vi "CAPTH Main Panel.vi"(11 "Expt State In":T2) -> (3 "Expt State Out":T2)   [LabVIEW 2020]
uses:
  CFTS Main Panel SubVIs/CFTS-Experiment State.ctl
  Typedefs/CAPTH-State.ctl
  CFTS Main Panel SubVIs/CFTS-Data Type Enum.ctl
panel:
  out "validate save history":bool
  out "XY Graph":cluster{"X":dbl, "Y":dbl}[](graph)
  out "finished":errorcluster
  in  "NOTES":string
  out "exit signal":bool
  in  "Analysis":bool
  in  "Response":T1={"Averages (3dB steps)"=12, "Time Window (ms)"=8.5, "dt (ms)"=10.0, "Grass gain"=1000.0, "CRITERION (uV)"=5.0, "CEILING (dB atten)"=6.0, "Use previous"=FALSE, "Save avgs"=FALSE, "Save raw"=FALSE, "Save history"=FALSE, "CEILING (dB SPL)"=6.0} {"CRITERION (uV)" format="%.2f"; "Time Window (ms)" format="%.2f"}
  out "User":string
  out "Run #":u16=14
  out "ID #":u16=1
  out "ave 2":cluster{i32, dbl, ext[]}(graph)={0, 0.01, []}
  in  "Stimulus":T3={" EAR"=enum."LEFT\n", "HI FREQ"=10.0, "LO FREQ"=2.5, "Steps/octave"=1, "Rep Rate (/s)"=20.0, "Alternate Polarity"=FALSE, "# CYCLES"=1, "Duration (ms)"=0.0, "Ramp (ms)"=0.0}
  in  "RETURN":bool
  in  "START":bool
  out "POST-EXPOSURE TIME (sec)":u32
  out "kHz":dbl=0.25 caption="Current frequency (kHz)" format="%.2f"
  out "Averages (1dB steps)":i32=24
  out "dB SPL 2":i32=20
  out "dB SPL 1":i32=74
  out "CYCLE":i32=1
  out "AUDIOGRAM":cluster{"Freq":dbl[], "Threshold":dbl[]}[](graph)
  out "ave 1":cluster{i32, dbl, ext[]}(graph)={0, 0.01, []}
  in  "STOP":bool
  # "Stimulus"
  # "1 dB per step"
  # "3 dB per step"
  # "Response"
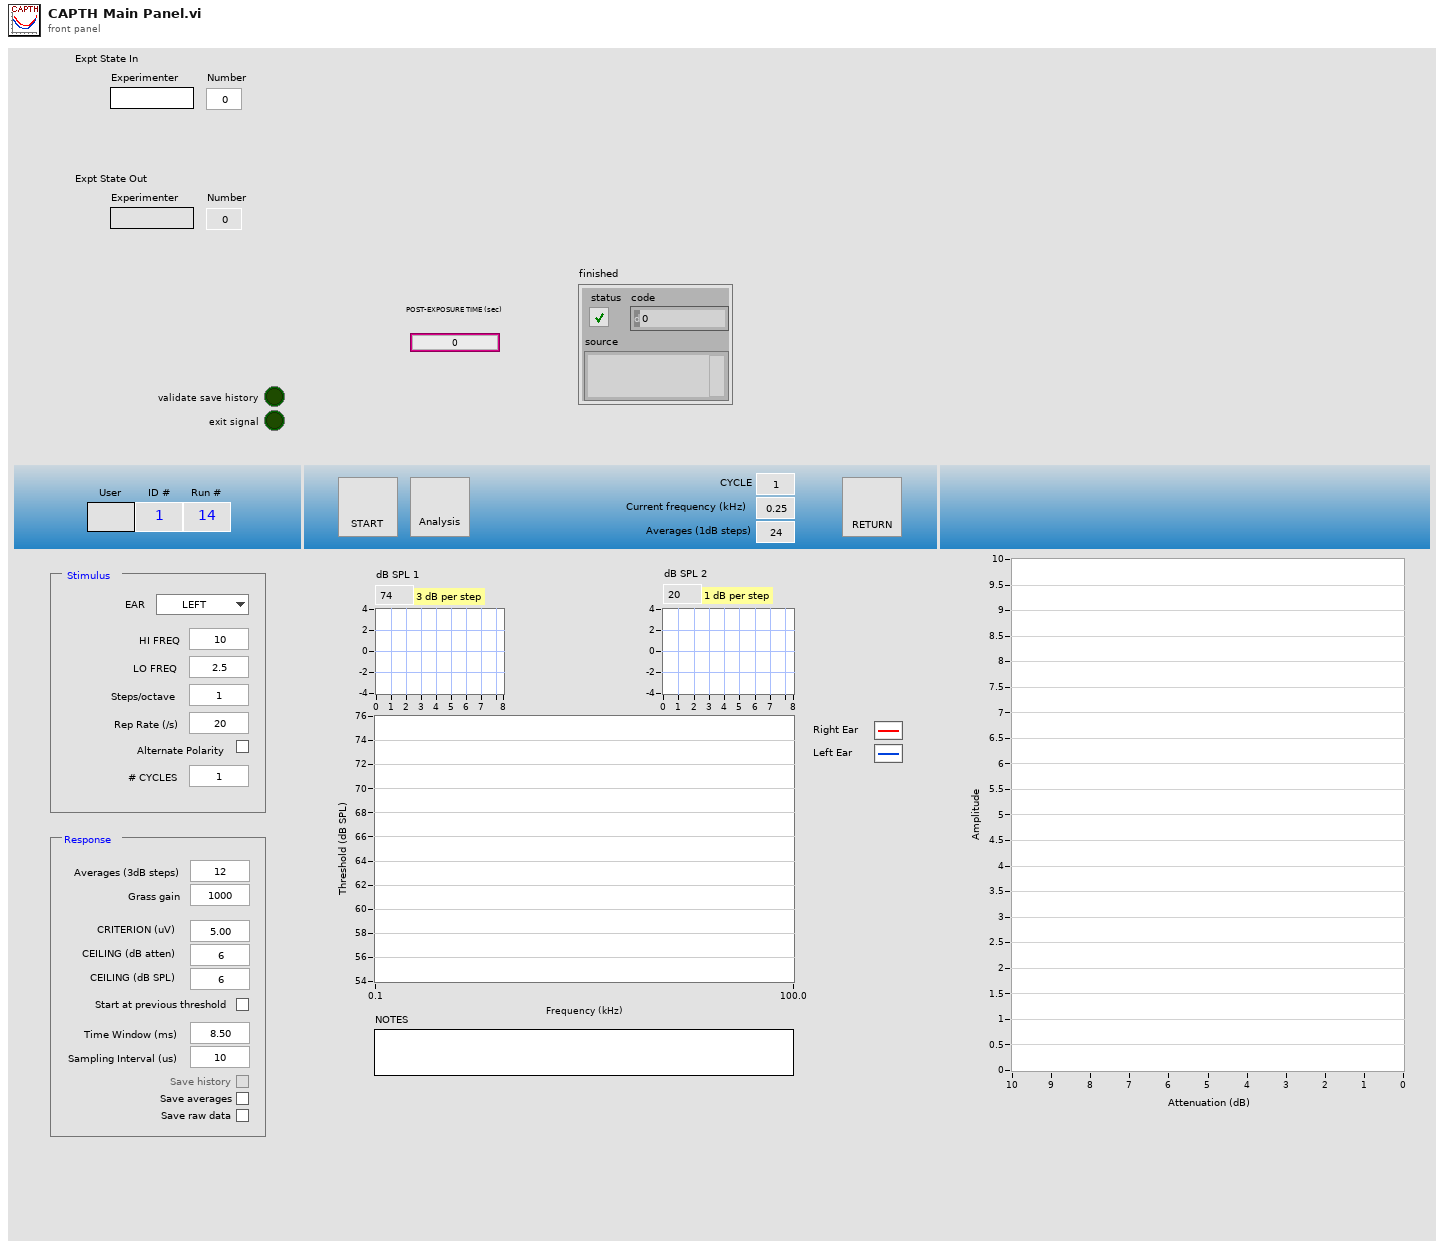
[diagram p1: front panel]
types:
  T1 = cluster{"Averages (3dB steps)":i32, "Time Window (ms)":dbl, "dt (ms)":dbl, "Grass gain":dbl, "CRITERION (uV)":dbl, "CEILING (dB atten)":dbl, "Use previous":bool, "Save avgs":bool, "Save raw":bool, "Save history":bool, "CEILING (dB SPL)":dbl}
  T2 = typedef "CFTS-Experiment State.ctl" = cluster{"Experimenter":string, "Number":u32, "Right":string, "Left":string, "Data Folder":path, "State File":path, "Version Info":string, "End Exposure Time":dbl, "Exposure Duration":string, "Run #":cluster{"CAP":i16, "ABR":i16, "DP":i16, "VsEP":i16, "MeasSeq":i16, "SubSeq":i16, "SFOAE":i16}}
  T3 = cluster{" EAR":enum16{"RIGHT", "LEFT\n", "ALTERNATE"}, "HI FREQ":dbl, "LO FREQ":dbl, "Steps/octave":u8, "Rep Rate (/s)":dbl, "Alternate Polarity":bool, "# CYCLES":u8, "Duration (ms)":dbl, "Ramp (ms)":dbl}
  T4 = typedef "CAPTH-IPC.ctl" = cluster{"Start":refnum<notifier>, "Control":refnum<notifier>, "Analysis":refnum<queue>}
  T5 = typedef "CAPTH-State.ctl" = cluster{"Datafile":path, "running":bool, "user":string, "aborted":bool}
  T6 = typedef "CFTS-Data Type Enum.ctl" = enum16{"CAP", "ABR", "DP", "VsEP", "MeasSeq", "SFOAE"}
  T7 = enum8{"Enabled", "Disabled", "Disabled and Grayed Out"}
  T8 = typedef "CAPTH-Parameters.ctl" = cluster{"Stimulus":T9, "Response":T10}
  T9 = typedef "CAPTH-Stimulus.ctl" = cluster{"EAR":enum16{"RIGHT", "LEFT\n", "ALTERNATE"}, "HI FREQ":dbl, "LO FREQ":dbl, "FREQ STEP":u8, "Rep Rate (/s)":dbl, "Alternate Polarity":bool, "# CYCLES":u8, "Duration (ms)":dbl, "Ramp (ms)":dbl}
  T10 = typedef "CAPTH-Response.ctl" = cluster{"Averages (3dB steps)":i32, "Time Window (ms)":dbl, "dt (us)":dbl, "Grass gain":dbl, "CRITERION (mV)":dbl, "CEILING (dB atten)":dbl, "Use previous":bool, "Save avgs":bool, "Save raw":bool, "Save history":bool, "CEILING (dB SPL)":dbl}
  T11 = cluster{"Freq":dbl[], "Threshold SPL":dbl[], "Max SPL":dbl[]}[]
  T12 = cluster{"Datafile path":path, "Params":T8, "data":cluster{"Freq":dbl[], "Threshold SPL":dbl[], "Max SPL":dbl[]}[]}
  T13 = typedef "CAPTH-Start Data.ctl" = cluster{"Datafile":path, "Params":T8, "data":cluster{"Freq":dbl[], "Threshold atten":dbl[], "Max SPL":dbl[]}[]}
  T14 = cluster{"Freq":dbl[], "Threshold atten":dbl[], "Max SPL":dbl[]}[]
  T15 = typedef "CAPTH-Runtime.ctl" = cluster{"Sampling rate":dbl, "AO npts":i32, "Alternate Polarity":bool, "AI npts":i32, "Npts window":i32, "1dB avgs":i32, "Datafile":path}
  T16 = typedef "CAPTH-StimCon.ctl" = cluster{"ear":i32, "freq":i32, "Max SPL":dbl}
  T17 = cluster{"Freq":dbl[], "Threshold":dbl[], "Max SPL":dbl[]}[]
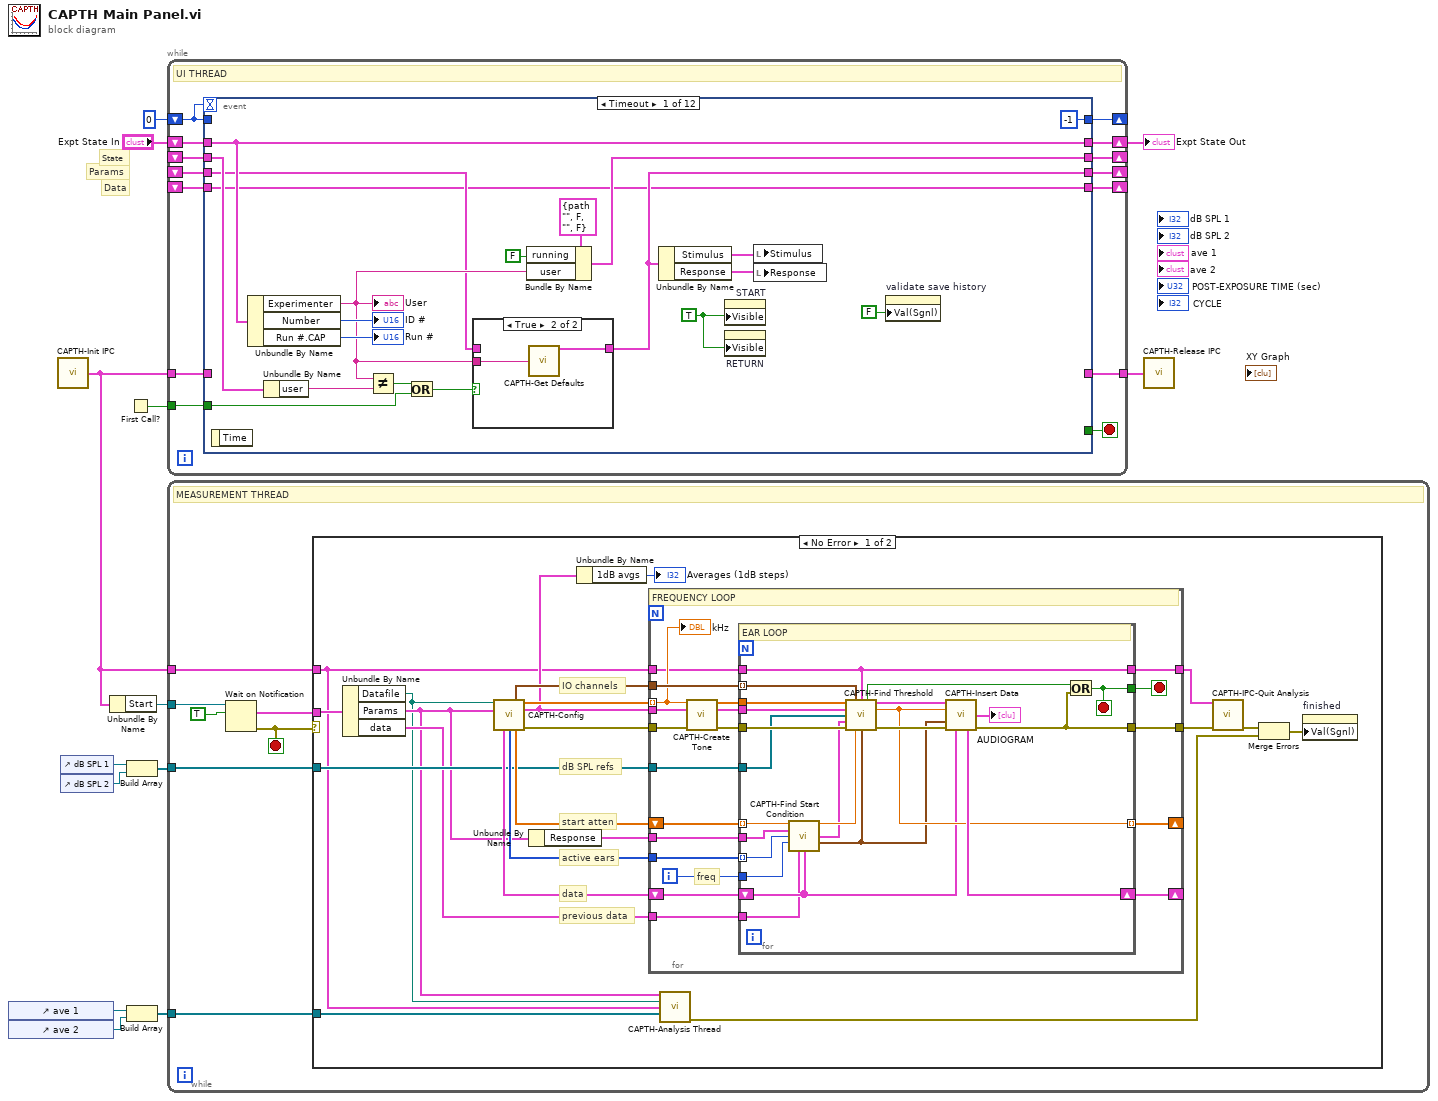
[diagram p0: block diagram]
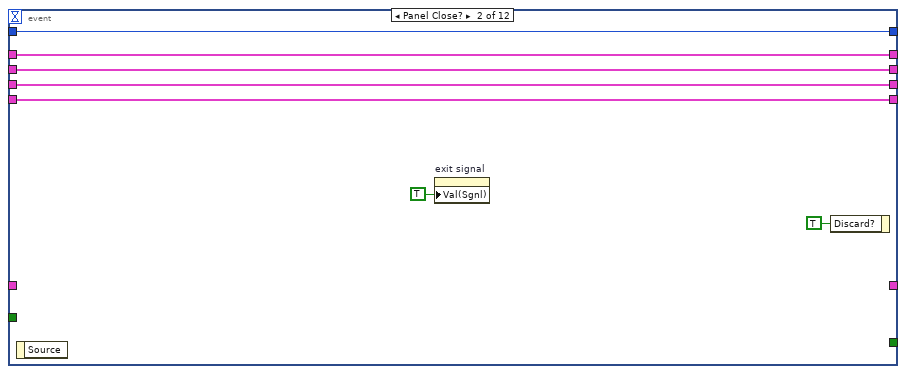
[diagram p4: hidden frame]
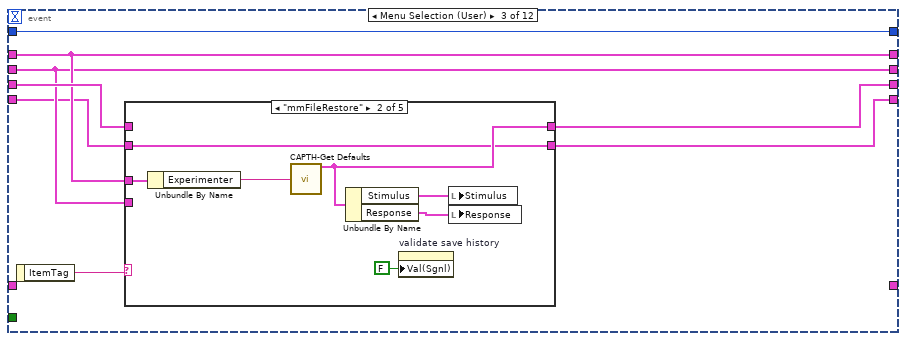
[diagram p5: hidden frame]
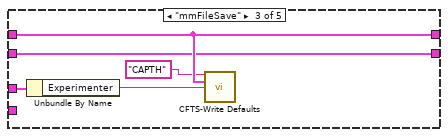
[diagram p7: hidden frame]
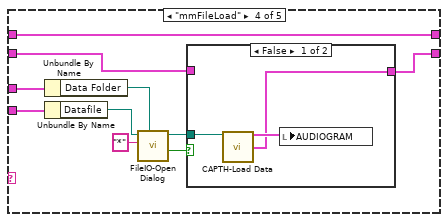
[diagram p8: hidden frame]
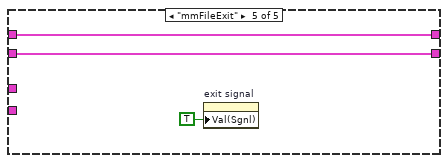
[diagram p10: hidden frame]
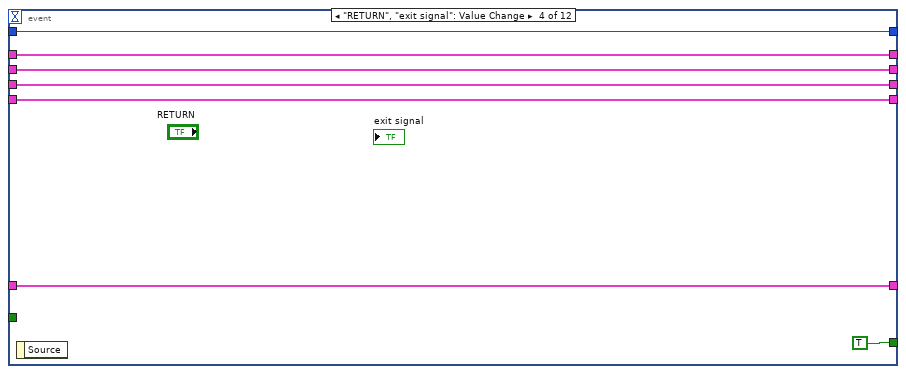
[diagram p11: hidden frame]
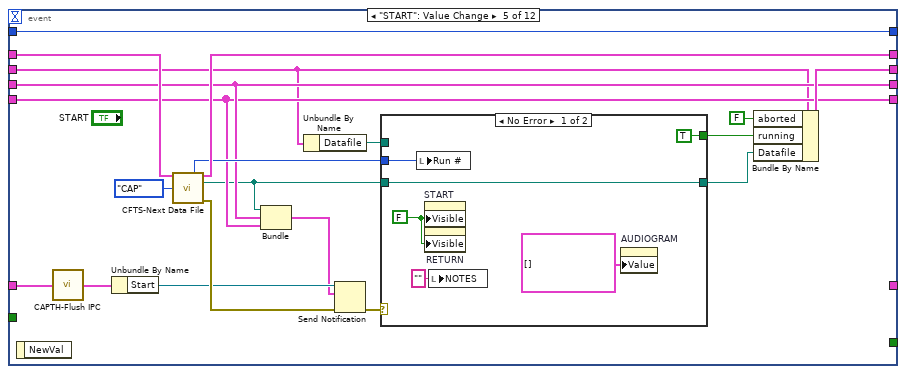
[diagram p12: hidden frame]
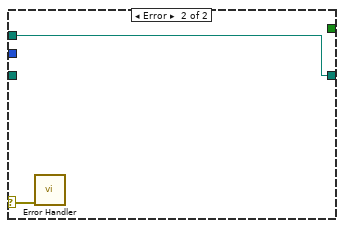
[diagram p13: hidden frame]
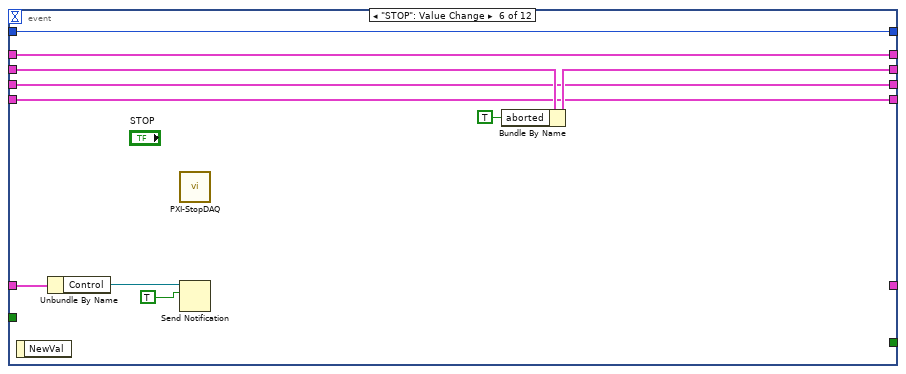
[diagram p14: hidden frame]
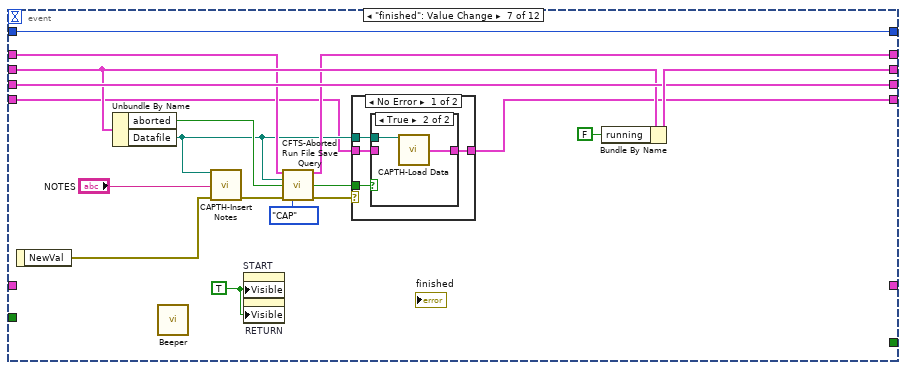
[diagram p15: hidden frame]
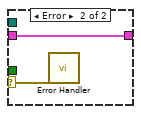
[diagram p17: hidden frame]
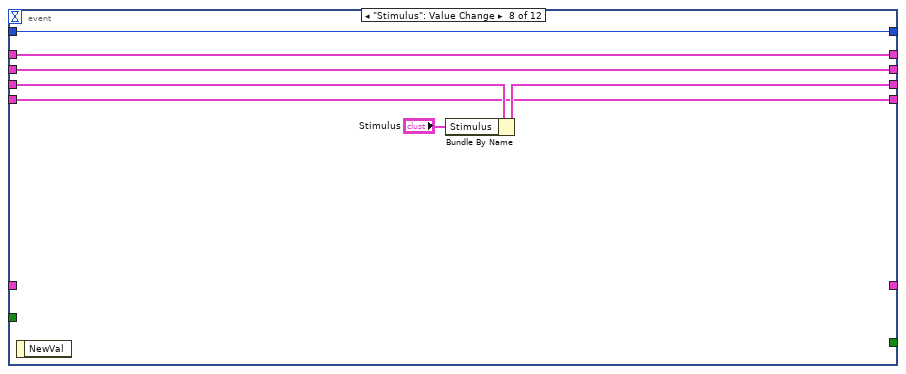
[diagram p18: hidden frame]
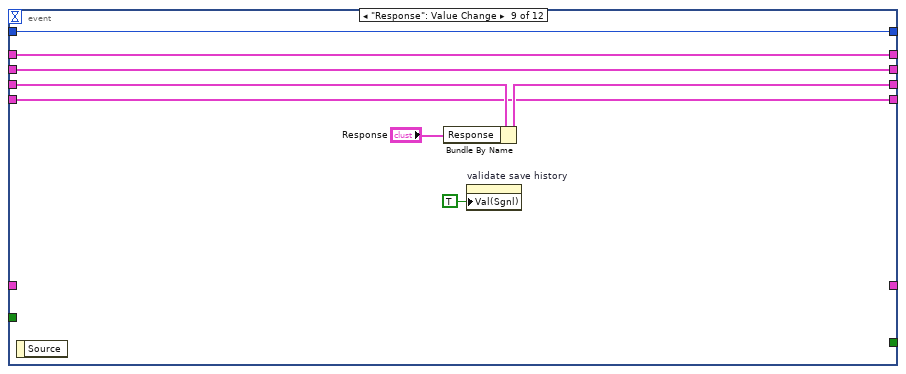
[diagram p19: hidden frame]
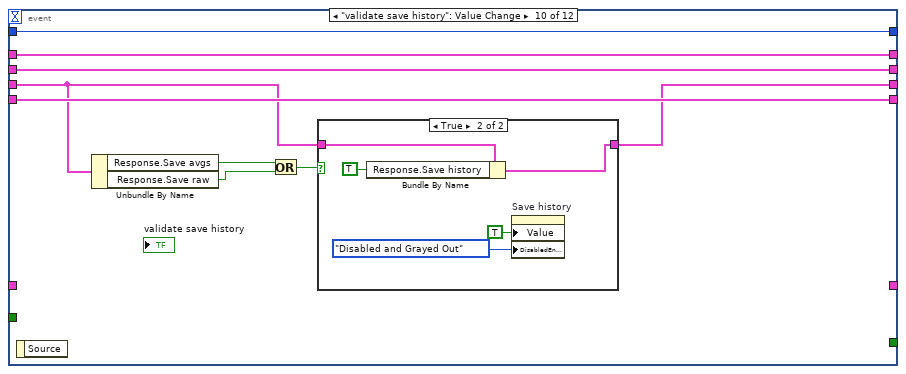
[diagram p20: hidden frame]
diagram:
  # "Data"
  # "Params"
  # "State"
  n1 = control-ref of="ave 1"() -> (w3:refnum<vi>)
  n2 = control-ref of="ave 2"() -> (w2:refnum<vi>)
  n3 = call "CAPTH-Init IPC.vi"() -> ("IPC"=w5:T4)  [unwired: 15 in]
  n4 = control-ref of="dB SPL 1"() -> (w10:refnum<vi>)
  n5 = control-ref of="dB SPL 2"() -> (w9:refnum<vi>)
  n6 = Unbundle By Name(w5) -> ("Start"=w7:refnum<notifier>)
  n7 = First Call?() -> (First Call?: T/F=w12:bool)
  n8 = Build Array(w10, w9) -> (w4:refnum<vi>[])
  n9 = Build Array(w3, w2) -> (w1:refnum<vi>[])
  n10 = while {
    tunnel: w5 -> [w27]
    shift-right: [w25] -> _
    shift-left: 0 -> [w21]
    tunnel: [w24] -> w6
    tunnel: w12 -> [w23]
    shift-right: [w20] -> w8
    shift-left: "Expt State In" -> [w22]
    shift-right: [w19] -> _
    shift-left: _ -> [w18]
    shift-right: [w16] -> _
    shift-left: _ -> [w17]
    shift-right: [w15] -> _
    shift-left: _ -> [w14]
    stop <- w26 stop-if-true
    # "UI THREAD"
    n11 = event shown="[0] Timeout" {
      selector: _ -> [_ _ _ _ _ _ _ _ _ _ _ _]
      dyn-events: _ -> [_ _ _ _ _ _ _ _ _ _ _ _]
      timeout: w21 -> [_ _ _ _ _ _ _ _ _ _ _ _]
      tunnel: w27 -> [_ _ _ w102 w109 w134 _ _ _ _ _ _]
      tunnel: [_ _ _ TRUE _ _ _ _ _ _ _ _] -> w26
      tunnel: [-1 w55 w64 w101 w123 w141 w159 w175 w183 w192 w206 w225] -> w25
      tunnel: [_ _ _ w102 _ _ _ _ _ _ _ _] -> w24
      tunnel: w23 -> [w41 _ _ _ _ _ _ _ _ _ _ _]
      tunnel: w22 -> [w40 w54 w61 w100 w119 w140 w147 w174 w182 w191 w205 w223]
      tunnel: w21 -> [_ w55 w64 w101 w123 w141 w159 w175 w183 w192 w206 w225]
      tunnel: [w40 w54 w61 w100 w118 w140 w146 w174 w182 w191 w205 w223] -> w20
      tunnel: [w39 w53 w60 w99 w122 w138 w157 w173 w181 w190 w204 w224] -> w19
      tunnel: w18 -> [w36 w53 w60 w99 w105 w139 w151 w173 w181 w190 w204 w224]
      tunnel: w17 -> [w33 w52 w62 w98 w113 w136 w155 w172 w180 w185 w202 w220]
      tunnel: [w32 w52 w63 w98 w113 w136 w155 w171 w179 w184 w202 w220] -> w16
      tunnel: [w29 w51 w59 w97 w112 w135 w144 w169 w177 w189 w201 w219] -> w15
      tunnel: w14 -> [w29 w51 w58 w97 w112 w135 w143 w169 w177 w189 w201 w219]
      event Timeout {
        w46 = TRUE ("Visible")
        n12 = event-data() -> ()  [unwired: 1 in, 1 out]
        n13 = Unbundle By Name(w40) -> ("Experimenter"=w37:string, "Number"=→"ID #":u32, "Run #.CAP"=→"Run #":i16)
        "User" <- w37
        n14 = Unbundle By Name(w36) -> ("user"=w35:string)
        n15 = Not Equal?(x=w37, y=w35) -> (x != y?=w43:bool)
        n16 = Or(x=w43, y=w41) -> (x .or. y?=w42:bool)
        n17 = case shown="True" w42 {
          tunnel: w37 -> [_ w49]
          tunnel: w33 -> [w48 _]
          tunnel: [w48 w50] -> w32
          frame False {
          }
          frame True {
            n18 = call "CAPTH-Get Defaults.vi"("User"=w49) -> ("Params"=w50:T8)  [unwired: 14 in]
          }
        }
        n19 = Bundle By Name(cluster=T5 {"Datafile"=path "", "running"=FALSE, "user"="", "aborted"=FALSE} ("State"), "running"=FALSE, "user"=w37) -> (w39:T5)
        n20 = Unbundle By Name(w32) -> ("Stimulus"=w31:T9, "Response"=w30:T10)
        n21 = property on="START" class="Bool"("Visible"=w46) -> ()  [unwired: 2 in, 2 out]
        n22 = property on="RETURN" class="Bool"("Visible"=w46) -> ()  [unwired: 2 in, 2 out]
        n23 = local write "Stimulus"(w31) -> ()
        n24 = local write "Response"(w30) -> ()
        n25 = property on="validate save history" class="Bool (strict)"("Val(Sgnl)"=FALSE ("Value (Signaling)")) -> ()  [unwired: 2 in, 2 out]
      }
      event Panel Close? {
        n26 = event-data() -> ()  [unwired: 1 in, 1 out]
        n27 = property on="exit signal" class="Bool (strict)"("Val(Sgnl)"=TRUE ("Value (Signaling)")) -> ()  [unwired: 2 in, 2 out]
        n28 = event-data("Discard?"=TRUE) -> ()  [unwired: 1 in, 1 out]
      }
      event Menu Selection (User) {
        n29 = event-data() -> ("ItemTag"=w65:string)  [unwired: 1 in]
        n30 = case shown="\"mmFileRestore\"" w65 {
          tunnel: w60 -> [_ _ _ w84 _]
          tunnel: [w67 w72 w77 w82 w95] -> w63
          tunnel: w62 -> [w67 _ w77 w82 w95]
          tunnel: w61 -> [_ w74 w79 w85 _]
          tunnel: [w66 w69 w75 w81 w94] -> w59
          tunnel: w58 -> [w66 w69 w75 w80 w94]
          frame "False", Default {
          }
          frame "mmFileRestore" {
            n31 = Unbundle By Name(w74) -> ("Experimenter"=w73:string)
            n32 = call "CAPTH-Get Defaults.vi"("User"=w73) -> ("Params"=w72:T8)  [unwired: 14 in]
            n33 = Unbundle By Name(w72) -> ("Stimulus"=w71:T9, "Response"=w70:T10)
            n34 = property on="validate save history" class="Bool (strict)"("Val(Sgnl)"=FALSE ("Value (Signaling)")) -> ()  [unwired: 2 in, 2 out]
            n35 = local write "Stimulus"(w71) -> ()
            n36 = local write "Response"(w70) -> ()
          }
          frame "mmFileSave" {
            n37 = Unbundle By Name(w79) -> ("Experimenter"=w78:string)
            n38 = call "CFTS-Write Defaults.vi"("AppName"="CAPTH", "Type of anything"=w77, "User"=w78) -> ()  [unwired: 11 in, 2 out]
          }
          frame "mmFileLoad" {
            n39 = Unbundle By Name(w85) -> ("Data Folder"=w89:path)
            n40 = Unbundle By Name(w84) -> ("Datafile"=w83:path)
            n41 = call "FileIO-Open Dialog.vi"("Default Folder"=w89, "pattern (all files)"="*", "Start path"=w83) -> ("cancelled"=w87:bool, "selected path"=w86:path)  [unwired: 6 in, 1 out]
            n42 = case shown="False" w87 {
              tunnel: w86 -> [w92 _]
              tunnel: [w90 w93] -> w81
              tunnel: w80 -> [_ w93]
              frame False {
                n43 = call "CAPTH-Load Data.vi"("Path"=w92) -> ("graph"=w91:cluster{dbl[], dbl[]}[], "data"=w90:T11)  [unwired: 13 in]
                n44 = local write "AUDIOGRAM"(w91) -> ()
              }
              frame True {
              }
            }
          }
          frame "mmFileExit" {
            n45 = property on="exit signal" class="Bool (strict)"("Val(Sgnl)"=TRUE ("Value (Signaling)")) -> ()  [unwired: 2 in, 2 out]
          }
        }
      }
      event "RETURN", "exit signal": Value Change {
        n46 = event-data() -> ()  [unwired: 1 in, 1 out]
      }
      event "START": Value Change {
        n47 = event-data() -> ()  [unwired: 1 in, 1 out]
        n48 = call "CAPTH-Flush IPC.vi"("IPC In"=w109) -> ("IPC Out"=w108:T4)  [unwired: 14 in]
        n49 = Unbundle By Name(w108) -> ("Start"=w111:refnum<notifier>)
        n50 = call "CFTS-Next Data File.vi"("Expt State"=w119, "Data Type"=CFTS-Data_Type_Enum."CAP") -> ("Run #"=w117:i16, "Expt State out"=w118:T2, "Datafile path"=w107:path, "error out"=w116:errorcluster)  [unwired: 9 in, 1 out]
        n51 = Bundle("Datafile path"=w107, "Params"=w113, "data"=w112) -> (w110:T12)  [unwired: 1 in]
        n52 = Unbundle By Name(w105) -> ("Datafile"=w104:path)
        n53 = Send Notification(notification=w110, notifier=w111, error in (no error)=w116) -> (error out=w115:errorcluster)  [unwired: 1 out]
        n54 = case shown="No Error" w115 {
          selector: w115 -> [_ w131]
          tunnel: w117 -> [w126 _]
          tunnel: [TRUE _] -> w114
          tunnel: w107 -> [w124 _]
          tunnel: [w124 w130] -> w106
          tunnel: w104 -> [_ w130]
          frame No Error {
            w129 = FALSE ("Visible")
            n55 = local write "Run #"(w126) -> ()
            n56 = property on="START" class="Bool"("Visible"=w129) -> ()  [unwired: 2 in, 2 out]
            n57 = property on="RETURN" class="Bool"("Visible"=w129) -> ()  [unwired: 2 in, 2 out]
            n58 = local write "NOTES"("" ("NOTES")) -> ()
            n59 = property on="AUDIOGRAM" class="XYGraph (strict)"("Value"=cluster{"Freq":dbl[], "Threshold":dbl[]}[] [] ("AUDIOGRAM")) -> ()  [unwired: 2 in, 2 out]
          }
          frame Error {
            n60 = call "Error Handler.vi"("error in (no error)"=w131) -> ()  [unwired: 13 in, 2 out]
          }
        }
        n61 = Bundle By Name(cluster=w105, "aborted"=FALSE, "running"=w114, "Datafile"=w106) -> (w122:T5)
      }
      event "STOP": Value Change {
        n62 = event-data() -> ()  [unwired: 1 in, 1 out]
        n63 = Unbundle By Name(w134) -> ("Control"=w133:refnum<notifier>)
        n64 = call "PXI-StopDAQ.vi"() -> ()  [unwired: 7 in, 1 out]
        n65 = Send Notification(notification=TRUE ("Stopping"), notifier=w133) -> ()  [unwired: 1 in, 2 out]
        n66 = Bundle By Name(cluster=w139, "aborted"=TRUE) -> (w138:T5)
      }
      event "finished": Value Change {
        w158 = TRUE ("Visible")
        n67 = event-data() -> ("NewVal"=w150:errorcluster)  [unwired: 1 in]
        n68 = Unbundle By Name(w151) -> ("aborted"=w148:bool, "Datafile"=w145:path)
        n69 = call "Beeper.vi"() -> ()  [unwired: 5 in, 1 out]
        n70 = call "CAPTH-Insert Notes.vi"("path"=w145, "Notes"="NOTES", "error in (no error)"=w150) -> ("error out"=w153:errorcluster)  [unwired: 12 in]
        n71 = property on="START" class="Bool"("Visible"=w158) -> ()  [unwired: 2 in, 2 out]
        n72 = property on="RETURN" class="Bool"("Visible"=w158) -> ()  [unwired: 2 in, 2 out]
        n73 = call "CFTS-Aborted Run File Save Query.vi"("Expt State"=w147, "Path"=w145, "Aborted"=w148, "error in (no error)"=w153, "Data Type"=CFTS-Data_Type_Enum."CAP") -> ("Expt State out"=w146:T2, "File saved?"=w142:bool, "error out"=w149:errorcluster)  [unwired: 8 in]
        n74 = case shown="No Error" w149 {
          selector: w149 -> [_ w168]
          tunnel: w145 -> [w163 _]
          tunnel: [w162 w167] -> w144
          tunnel: w143 -> [w160 w167]
          tunnel: w142 -> [w161 _]
          frame No Error {
            n75 = case shown="True" w161 {
              tunnel: w163 -> [_ w166]
              tunnel: [w164 w165] -> w162
              tunnel: w160 -> [w164 _]
              frame False {
              }
              frame True {
                n76 = call "CAPTH-Load Data.vi"("Path"=w166) -> ("data"=w165:T11)  [unwired: 13 in, 1 out]
              }
            }
          }
          frame Error {
            n77 = call "Error Handler.vi"("error in (no error)"=w168) -> ()  [unwired: 13 in, 2 out]
          }
        }
        n78 = Bundle By Name(cluster=w151, "running"=FALSE) -> (w157:T5)
      }
      event "Stimulus": Value Change {
        n79 = event-data() -> ()  [unwired: 1 in, 1 out]
        n80 = Bundle By Name(cluster=w172, "Stimulus"="Stimulus") -> (w171:T8)
      }
      event "Response": Value Change {
        n81 = event-data() -> ()  [unwired: 1 in, 1 out]
        n82 = Bundle By Name(cluster=w180, "Response"="Response") -> (w179:T8)
        n83 = property on="validate save history" class="Bool (strict)"("Val(Sgnl)"=TRUE ("Value (Signaling)")) -> ()  [unwired: 2 in, 2 out]
      }
      event "validate save history": Value Change {
        n84 = event-data() -> ()  [unwired: 1 in, 1 out]
        n85 = Unbundle By Name(w185) -> ("Response.Save avgs"=w187:bool, "Response.Save raw"=w186:bool)
        n86 = Or(x=w187, y=w186) -> (x .or. y?=w188:bool)
        n87 = case shown="True" w188 {
          tunnel: w185 -> [w193 w197]
          tunnel: [w193 w195] -> w184
          frame False {
            n88 = property on="Save history" class="Bool (strict)"("DisabledEnum"=T7."Enabled" ("Disabled")) -> ()  [unwired: 2 in, 2 out]
          }
          frame True {
            n89 = Bundle By Name(cluster=w197, "Response.Save history"=TRUE) -> (w195:T8)
            n90 = property on="Save history" class="Bool (strict)"("Value"=TRUE, "DisabledEnum"=T7."Disabled and Grayed Out" ("Disabled")) -> ()  [unwired: 2 in, 2 out]
          }
        }
      }
      event "NOTES": Value Change {
        n91 = event-data() -> ("NewVal"=w208:string)  [unwired: 1 in]
        n92 = Unbundle By Name(w204) -> ("Datafile"=w200:path, "running"=w203:bool)
        n93 = Not(x=w203) -> (.not. x?=w211:bool)
        n94 = Empty String/Path?(string/path=w200) -> (empty?=w212:bool)
        n95 = Not(x=w212) -> (.not. x?=w210:bool)
        n96 = And(x=w210, y=w211) -> (x .and. y?=w209:bool)
        n97 = case shown="True" w209 {
          tunnel: w200 -> [_ w216]
          tunnel: w208 -> [_ w215]
          tunnel: "Add notes to data file?" ("message") -> [_ w214]
          frame False {
          }
          frame True {
            n98 = Two Button Dialog(message=w214) -> (T button?=w213:bool)  [unwired: 2 in]
            n99 = case shown="True" w213 {
              tunnel: w216 -> [_ w218]
              tunnel: w215 -> [_ w217]
              frame False {
              }
              frame True {
                n100 = call "CAPTH-Insert Notes.vi"("path"=w218, "Notes"=w217) -> ()  [unwired: 13 in, 1 out]
              }
            }
          }
        }
      }
      event "Analysis": Value Change {
        n101 = event-data() -> ()  [unwired: 1 in, 1 out]
        n102 = Unbundle By Name(w223) -> ("Experimenter"=w222:string, "Number"=w221:u32)
        n103 = call "CAPTH-Simulplot.vi"("ID"=w221, "User"=w222) -> ()  [unwired: 10 in]
      }
    }
  }
  "Expt State Out" <- w8
  n104 = while {
    tunnel: w7 -> [w231]
    tunnel: w4 -> [w229]
    tunnel: w5 -> [w227]
    tunnel: w1 -> [w226]
    stop <- w230 stop-if-true
    # "MEASUREMENT THREAD"
    n105 = Wait on Notification(notifier=w231, ignore previous (F)=TRUE) -> (notification=w228:T13, error out=w230:errorcluster)  [unwired: 2 in, 2 out]
    n106 = case shown="No Error" w230 {
      tunnel: w229 -> [w246 _]
      tunnel: w228 -> [w245 _]
      tunnel: w227 -> [w238 _]
      tunnel: w226 -> [w239 _]
      frame No Error {
        # "previous data"
        # "dB SPL refs"
        # "start atten"
        # "IO channels"
        # "active ears"
        # "data"
        n107 = Unbundle By Name(w245) -> ("Datafile"=w240:path, "Params"=w241:T8, "data"=w244:T14)
        n108 = call "CAPTH-Config.vi"("Datafile"=w240, "Params"=w241) -> ("IO channels"=w250:cluster{"Output":u16, "Input":u16}[], "Freqs"=w249:dbl[], "runtime"=w242:T15, "data"=w252:T14, "active ears"=w251:i32[], "start atten"=w248:dbl[], "error out"=w253:errorcluster)  [unwired: 7 in]
        n109 = Unbundle By Name(w241) -> ("Response"=w243:T10)
        n110 = Unbundle By Name(w242) -> ("1dB avgs"=→"Averages (1dB steps)":i32)
        n111 = for {
          tunnel: w242 -> [w264]
          tunnel: w253 -> [w273]
          tunnel: [w260] -> w235
          shift-right: [w269] -> _
          shift-left: w252 -> [w270]
          tunnel: w251 -> [w268]
          tunnel: w250 -> [w267]
          shift-right: [w266] -> _
          shift-left: w248 -> [w263]
          tunnel: w249 -> [w265] mode=indexing
          tunnel: w244 -> [w258]
          tunnel: w246 -> [w257]
          tunnel: w243 -> [w256]
          tunnel: w238 -> [w255]
          tunnel: [w254] -> w233
          i -> [w271]
          stop <- w259 stop-if-true
          # "freq"
          # "FREQUENCY LOOP"
          n112 = call "CAPTH-Create Tone.vi"("Freq (kHz)"=w265, "runtime in"=w264, "error in (no error)"=w273) -> ("tone"=w262:dbl[], "runtime out"=w261:T15, "error out"=w272:errorcluster)  [unwired: 10 in]
          n113 = for {
            tunnel: w272 -> [w296]
            tunnel: [w280] -> w260
            tunnel: w271 -> [w278]
            shift-right: [w293] -> w269
            shift-left: w270 -> [w288]
            tunnel: w268 -> [w277] mode=indexing
            tunnel: w267 -> [w294] mode=indexing
            tunnel: [w289] -> w266 mode=indexing
            tunnel: w263 -> [w287] mode=indexing
            tunnel: w262 -> [w292]
            tunnel: w261 -> [w290]
            tunnel: [w281] -> w259
            tunnel: w258 -> [w285]
            tunnel: w257 -> [w284]
            tunnel: w256 -> [w283]
            tunnel: w255 -> [w275]
            tunnel: [w275] -> w254
            stop <- w281 stop-if-true
            # "EAR LOOP"
            n114 = call "CAPTH-Find Start Condition.vi"("nominal start atten"=w287, "Response in"=w283, "ear"=w277, "freq"=w278, "last data"=w285, "data"=w288) -> ("start atten"=w286:dbl, "Response out"=w274:T10, "stimcon"=w276:T16)  [unwired: 6 in, 1 out]
            n115 = call "CAPTH-Find Threshold.vi"("tone"=w292, "Channels"=w294, "IPC"=w275, "runtime"=w290, "dB refs"=w284, "Response"=w274, "error in (no error)"=w296, "Start atten"=w286, "stimcon"=w276) -> ("Abort"=w279:bool, "runtime out"=w282:T15, "Threshold"=w289:dbl, "error out"=w295:errorcluster)  [unwired: 3 in]
            n116 = call "CAPTH-Insert Data.vi"("Runtime"=w282, "Threshold"=w289, "stimcon"=w276, "error in (no error)"=w295, "data"=w288) -> ("Plot Array"=→"AUDIOGRAM":cluster{"Freq":dbl[], "Threshold":dbl[]}[], "data out"=w293:T17, "error out"=w280:errorcluster)  [unwired: 8 in]
            n117 = Or(x=w279, y=w280) -> (x .or. y?=w281:bool)
          }
          "kHz" <- w265
        }
        n118 = call "CAPTH-Analysis Thread.vi"("Params"=w241, "Datafile"=w240, "IPC"=w238, "avg refs"=w239) -> ("error out"=w236:errorcluster)  [unwired: 11 in]
        n119 = call "CAPTH-IPC-Quit Analysis.vi"("IPC"=w233, "error in (no error)"=w235) -> ("error out"=w234:errorcluster)  [unwired: 13 in]
        n120 = Merge Errors(w234, w236) -> (w237:errorcluster)
        n121 = property on="finished" class="Clust (strict)"("Val(Sgnl)"=w237) -> ()  [unwired: 2 in, 2 out]
      }
      frame Error {
      }
    }
  }
  n122 = call "CAPTH-Release IPC.vi"("IPC"=w6) -> ()  [unwired: 15 in]
